vi "WPI_CameraClose.vi"(8 "error in (no error)":errorcluster, 11 "CameraDevRef":T1) -> (0 "error out":errorcluster)   [LabVIEW 2017]
doc: "Closes the reference to the camera, stops acquiring image data, and stops sending image data to the host computer. If the count of the camera reference is greater than one, this VI only decrements the count of the camera reference by one.\n\nThis software is licensed. Open the labview\\readme\\WPI Robotics Library Open Source License.txt file for more information."
uses:
  <vilib>/Rock Robotics/WPI/Camera/WPI_CameraDevRef.ctl
  <vilib>/Rock Robotics/WPI/Camera/WPI_CameraRegistryActions.ctl
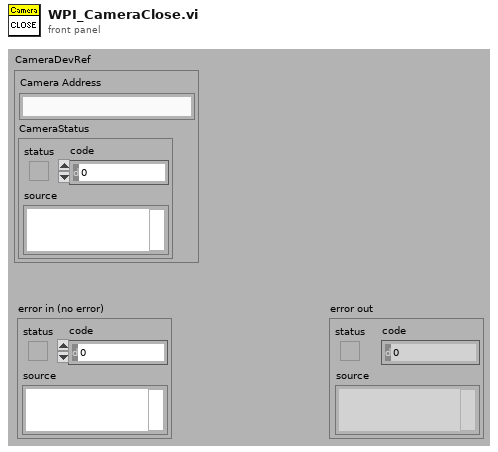
[diagram p1: front panel]
types:
  T1 = typedef "WPI_CameraDevRef.ctl" = cluster{"Camera Address":string, "CameraStatus":errorcluster}
  T2 = typedef "WPI_CameraRegistryActions.ctl" = enum16{"Open", "Close"}
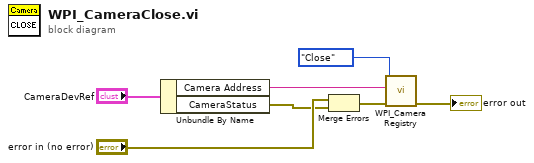
[diagram p0: block diagram]
diagram:
  n1 = Unbundle By Name("CameraDevRef") -> ("Camera Address"=w6:string, "CameraStatus"=w2:errorcluster)
  n2 = Merge Errors("error in (no error)", w2) -> (w1:errorcluster)
  n3 = call <vilib>:"WPI_Camera Registry.vi"("error in (no error)"=w1, "Camera Address"=w6, "Action"=WPI_CameraRegistryActions."Close" ("Enum")) -> ("error out"=→"error out":errorcluster)  [unwired: 8 out]
